vi "Set Output Node Enable.vi"(6 "Update":bool=TRUE, 7 "Enable":i32, 8 "error in (no error)":errorcluster, 9 "node":i32, 10 "idxChannel":i32, 11 "hdwf":i32) -> (0 "error out":errorcluster, 1 "func_out":i32)   [LabVIEW 2024, in "AD2 DLL.lvlib"]
uses:
  AD2 DLL.lvlib
  <vilib>/Digilent/AD2 Toolkit/AD2.lvlib
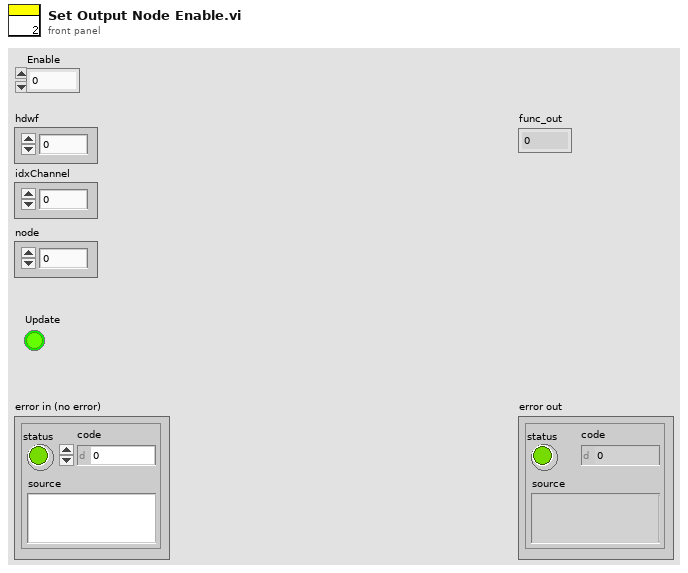
[diagram p1: front panel]
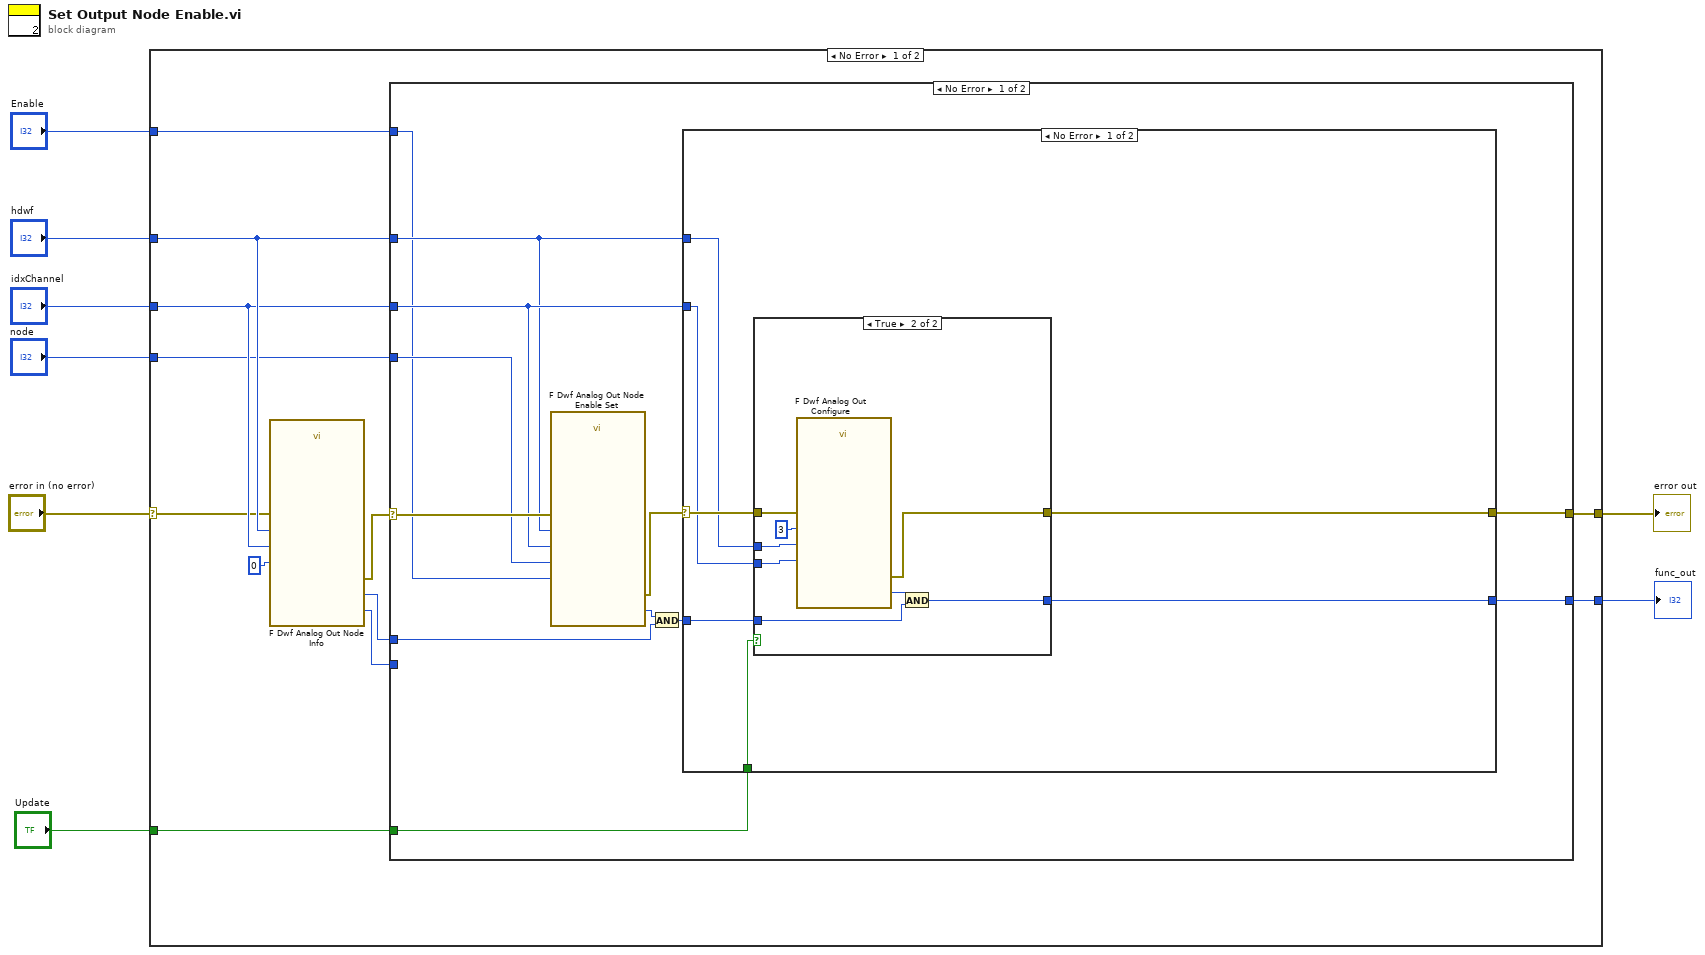
[diagram p0: block diagram]
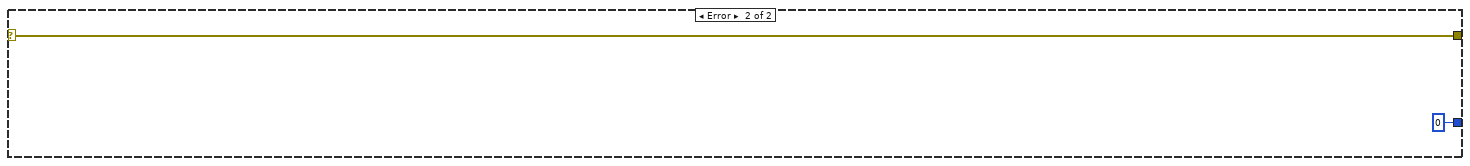
[diagram p5: hidden frame]
diagram:
  n1 = case shown="No Error" "error in (no error)" {
    selector: "error in (no error)" -> [w11 w55]
    tunnel: [w19 w55] -> w8
    tunnel: "hdwf" -> [w14 _]
    tunnel: "idxChannel" -> [w13 _]
    tunnel: "node" -> [w12 _]
    tunnel: "Enable" -> [w20 _]
    tunnel: [w18 0] -> w2
    tunnel: "Update" -> [w17 _]
    frame No Error {
      n2 = call <vilib>:"F Dwf Analog Out Node Info.vi"("error in (no error)"=w11, "pfsnode"=0, "idxChannel"=w13, "hdwf"=w14) -> ("error out"=w16:errorcluster, "pfsnode out"=w10:i32, "function return"=w15:i32)  [unwired: 5 in]
      n3 = case shown="No Error" w16 {
        selector: w16 -> [w25 w53]
        tunnel: w20 -> [w21 _]
        tunnel: [w32 w53] -> w19
        tunnel: w14 -> [w22 _]
        tunnel: w13 -> [w24 _]
        tunnel: w12 -> [w23 _]
        tunnel: w15 -> [w31 w52]
        tunnel: [w29 w52] -> w18
        tunnel: w17 -> [w28 _]
        tunnel: w10 -> [_ _]
        frame No Error {
          n4 = call <vilib>:"F Dwf Analog Out Node Enable Set.vi"("fEnable"=w21, "error in (no error)"=w25, "node"=w23, "idxChannel"=w24, "hdwf"=w22) -> ("error out"=w27:errorcluster, "function return"=w26:i32)  [unwired: 5 in]
          n5 = And(x=w26, y=w31) -> (x .and. y?=w30:i32)
          n6 = case shown="No Error" w27 {
            selector: w27 -> [w39 w51]
            tunnel: [w36 w51] -> w32
            tunnel: w22 -> [w38 _]
            tunnel: w24 -> [w37 _]
            tunnel: w30 -> [w35 w50]
            tunnel: [w34 w50] -> w29
            tunnel: w28 -> [w33 _]
            frame No Error {
              n7 = case shown="True" w33 {
                tunnel: w39 -> [w41 w49]
                tunnel: w38 -> [_ w47]
                tunnel: w37 -> [_ w46]
                tunnel: [w41 w45] -> w36
                tunnel: w35 -> [w40 w43]
                tunnel: [w40 w42] -> w34
                frame False {
                }
                frame True {
                  n8 = call <vilib>:"F Dwf Analog Out Configure.vi"("error in (no error)"=w49, "fStart"=3, "idxChannel"=w46, "hdwf"=w47) -> ("error out"=w45:errorcluster, "function return"=w44:i32)  [unwired: 6 in]
                  n9 = And(x=w44, y=w43) -> (x .and. y?=w42:i32)
                }
              }
            }
            frame Error {
            }
          }
        }
        frame Error {
        }
      }
    }
    frame Error {
    }
  }
  "error out" <- w8
  "func_out" <- w2
